vi "Radial Coefficient Calc.vi"(1 "T2":dbl, 2 "T1":dbl, 3 "Power":dbl, 4 "Thikness":dbl, 5 "ri":dbl, 6 "ro":dbl) -> (0 "K":dbl)   [LabVIEW 2017]
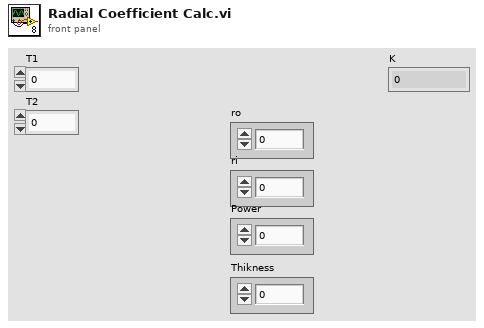
[diagram p1: front panel]
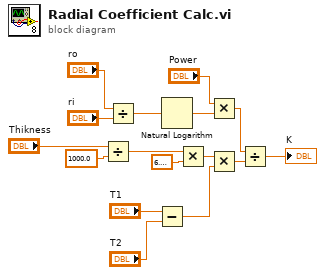
[diagram p0: block diagram]
diagram:
  n1 = Divide(x="Thikness", y=1000.0) -> (x/y=w2:dbl)
  n2 = Divide(x="ro", y="ri") -> (x/y=w14:dbl)
  n3 = Subtract(x="T1", y="T2") -> (x-y=w7:dbl)
  n4 = Natural Logarithm(1:w14) -> (0:w13:dbl)
  n5 = Multiply(x=w2, y=6.283185307179586) -> (x*y=w8:dbl)
  n6 = Multiply(x="Power", y=w13) -> (x*y=w11:dbl)
  n7 = Multiply(x=w8, y=w7) -> (x*y=w6:dbl)
  n8 = Divide(x=w11, y=w6) -> (x/y=→"K":dbl)
